vi "Generate Channels.vi"(8 "error in (no error)":errorcluster, 11 "Lakeshore 331 in":refnum<class "Lakeshore 331.lvclass">) -> (0 "error out":errorcluster, 1 "Channel Names":string[](array[string])=["Telescope RA", "Telescope DEC", "Telescope Moving?", "Telescope Status"], 2 "Channel List":refnum<class "HK Item.lvclass">[](array[class]), 3 "Lakeshore 331 out":refnum<class "Lakeshore 331.lvclass">)   [LabVIEW 2022 SP3, in "Lakeshore 331.lvclass"]
uses:
  Lakeshore 331.lvclass
  hk-channel-class/hk-channel-class/HK Item/HK Item.lvclass
  Lakeshore 331.lvclass/Lakeshore 331.ctl
  Temp Control.lvclass
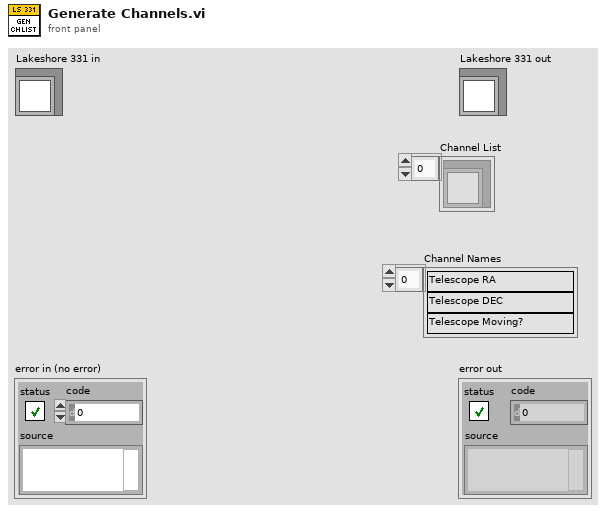
[diagram p1: front panel]
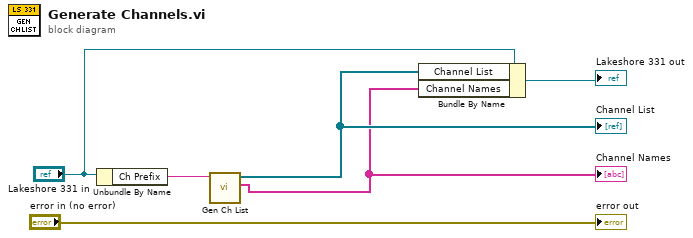
[diagram p0: block diagram]
diagram:
  n1 = Unbundle By Name("Lakeshore 331 in") -> ("Ch Prefix"=w6:string)
  n2 = call "Gen Ch List.vi"("Prefix"=w6) -> ("Channel Names"=w2:string[], "Channel List"=w3:refnum<class "HK Item.lvclass">[])  [unwired: 9 in]
  "Channel List" <- w3
  "Channel Names" <- w2
  n3 = Bundle By Name(cluster="Lakeshore 331 in", "Channel List"=w3, "Channel Names"=w2) -> (→"Lakeshore 331 out":refnum<class "Lakeshore 331.lvclass">)
  "error out" <- "error in (no error)"
